vi "FGV_ROI.vi"(7 "Action_ROI":T3, 8 "Error in":errorcluster, 10 "ROI Name":string, 11 "ROI In":T1 {"Contours"."Type" items=["No Selection", "Point", "Line", "Rectangle", "Oval", "Polygon", "Free", "Annulus", "Unused2", "Unused3", "Broken Line", "Free Hand Line", "Rotated Rectangle"]}) -> (0 "Error out":errorcluster, 1 "ROI Array":T2(array[cluster]) {"Contours"."Type" items=["No Selection", "Point", "Line", "Rectangle", "Oval", "Polygon", "Free", "Annulus", "Unused2", "Unused3", "Broken Line", "Free Hand Line", "Rotated Rectangle"]}, 2 "ROI Name Array":string[](array[string]), 3 "ROI Out":T1 {"Contours"."Type" items=["No Selection", "Point", "Line", "Rectangle", "Oval", "Polygon", "Free", "Annulus", "Unused2", "Unused3", "Broken Line", "Free Hand Line", "Rotated Rectangle"]})   [LabVIEW 2015]
uses:
  <userlib>/FGV/control/Control_ROI.ctl
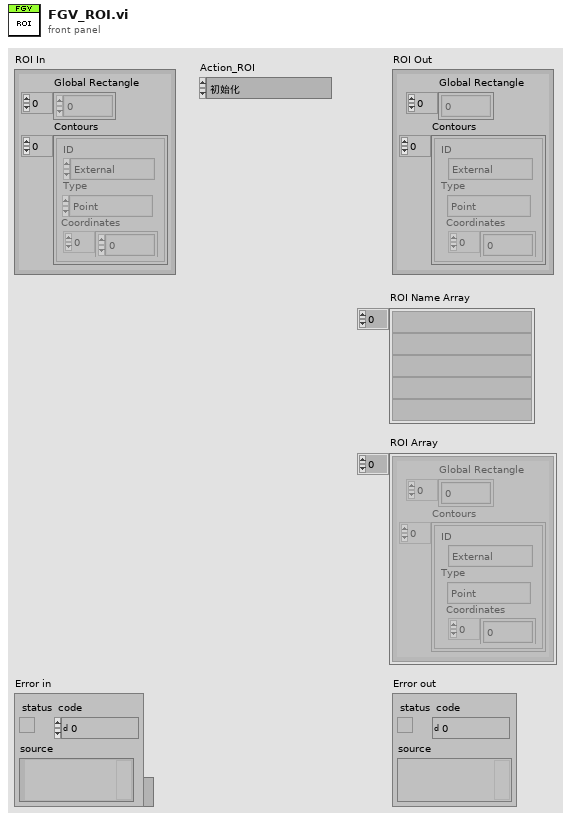
[diagram p1: front panel]
types:
  T1 = cluster{"Global Rectangle":i32[], "Contours":cluster{"ID":enum32{"External", "Internal"}, "Type":u32, "Coordinates":i32[]}[]}
  T2 = cluster{"Global Rectangle":i32[], "Contours":cluster{"ID":enum32{"External", "Internal"}, "Type":u32, "Coordinates":i32[]}[]}[]
  T3 = typedef "Control_ROI.ctl" = enum16{"初始化", "建立ROI", "寫入ROI", "讀出ROI", "刪除ROI"}
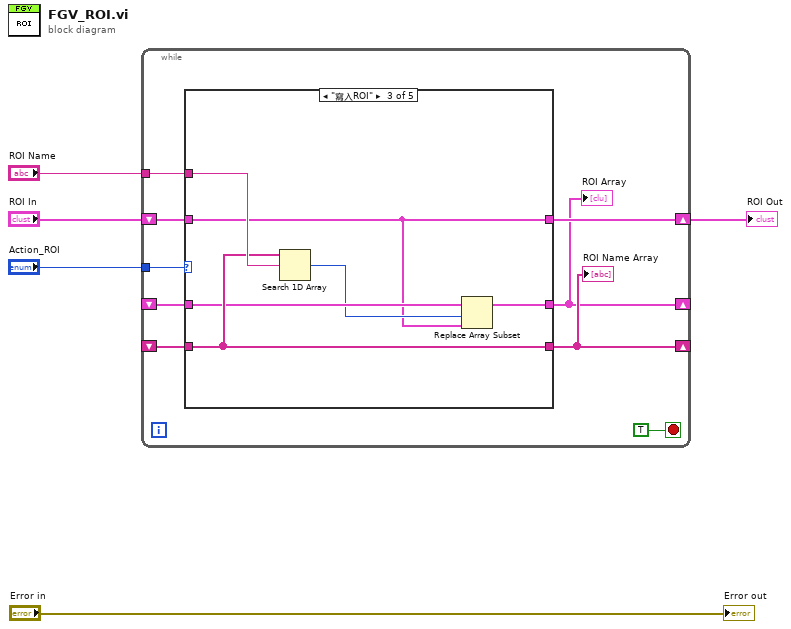
[diagram p0: block diagram]
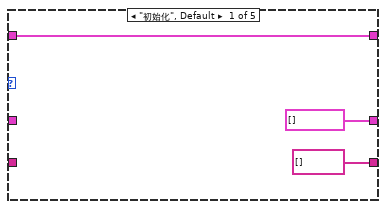
[diagram p2: hidden frame]
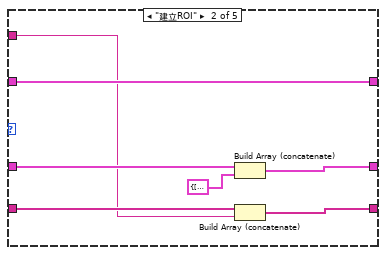
[diagram p3: hidden frame]
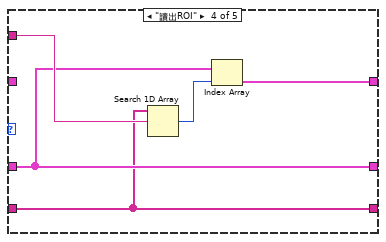
[diagram p4: hidden frame]
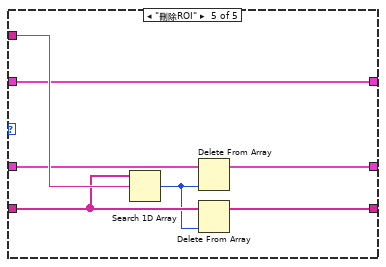
[diagram p5: hidden frame]
diagram:
  n1 = while {
    tunnel: "Action_ROI" -> [w13]
    tunnel: "ROI Name" -> [w12]
    shift-right: [w11] -> w3
    shift-left: "ROI In" -> [w10]
    shift-right: [w6] -> _
    shift-left: _ -> [w9]
    shift-right: [w7] -> _
    shift-left: _ -> [w8]
    stop <- TRUE stop-if-true
    n2 = case shown="\"寫入ROI\"" w13 {
      tunnel: w12 -> [_ w19 w30 w35 w42]
      tunnel: [w17 w20 w25 w33 w36] -> w11
      tunnel: w10 -> [w17 w20 w25 _ w36]
      tunnel: [T2 [] ("ROI Array") w23 w27 w32 w38] -> w6
      tunnel: w9 -> [_ w24 w28 w32 w41]
      tunnel: [string[] [] w21 w29 w31 w37] -> w7
      tunnel: w8 -> [_ w22 w29 w31 w40]
      frame "初始化", Default {
      }
      frame "建立ROI" {
        n3 = Build Array (concatenate)(w24, T1 {"Global Rectangle"=[0, 0, 0, 0], "Contours"=[{"ID"=enum."External", "Type"=1, "Coordinates"=[0, 0, 0, 0, 0, 0]}]} ("ROI")) -> (w23:T2)
        n4 = Build Array (concatenate)(w22, w19) -> (w21:string[])
      }
      frame "寫入ROI" {
        n5 = Search 1D Array(1D array=w29, element=w30) -> (index of element=w26:i32)  [unwired: 1 in]
        n6 = Replace Array Subset(array=w28, new element=w25, index=w26) -> (w27:T2)
      }
      frame "讀出ROI" {
        n7 = Search 1D Array(1D array=w31, element=w35) -> (index of element=w34:i32)  [unwired: 1 in]
        n8 = Index Array(array=w32, index=w34) -> (element=w33:T1)
      }
      frame "刪除ROI" {
        n9 = Search 1D Array(1D array=w40, element=w42) -> (index of element=w39:i32)  [unwired: 1 in]
        n10 = Delete From Array(array=w41, index=w39) -> (array with subset deleted=w38:T2)  [unwired: 1 in, 1 out]
        n11 = Delete From Array(array=w40, index=w39) -> (array with subset deleted=w37:string[])  [unwired: 1 in, 1 out]
      }
    }
    "ROI Name Array" <- w7
    "ROI Array" <- w6
  }
  "ROI Out" <- w3
  "Error out" <- "Error in"
